vi "Cron&EventTab@ShortcutsStart__Parameter.vi"(1 "ParamterIn":string) -> (0 "ParamterOut":string)   [LabVIEW 2020]
panel:
  in  "Conditioin":string
  in  "EventTabName":string(combo)
  in  "Confirm":bool
  # "Cron&EventTab@ShortcutsStart $ShortcutsTabName, $Key"
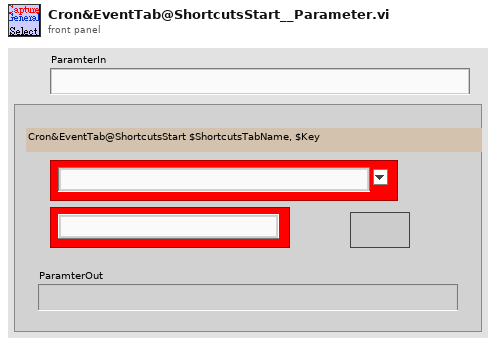
[diagram p1: front panel]
types:
  T1 = enum16{"Init", "Add", "Enable", "Disable", "Get"}
  T2 = cluster{"Shift":bool, "Ctrl":bool, "Alt":bool, "Cmd":bool, "Opt":bool}
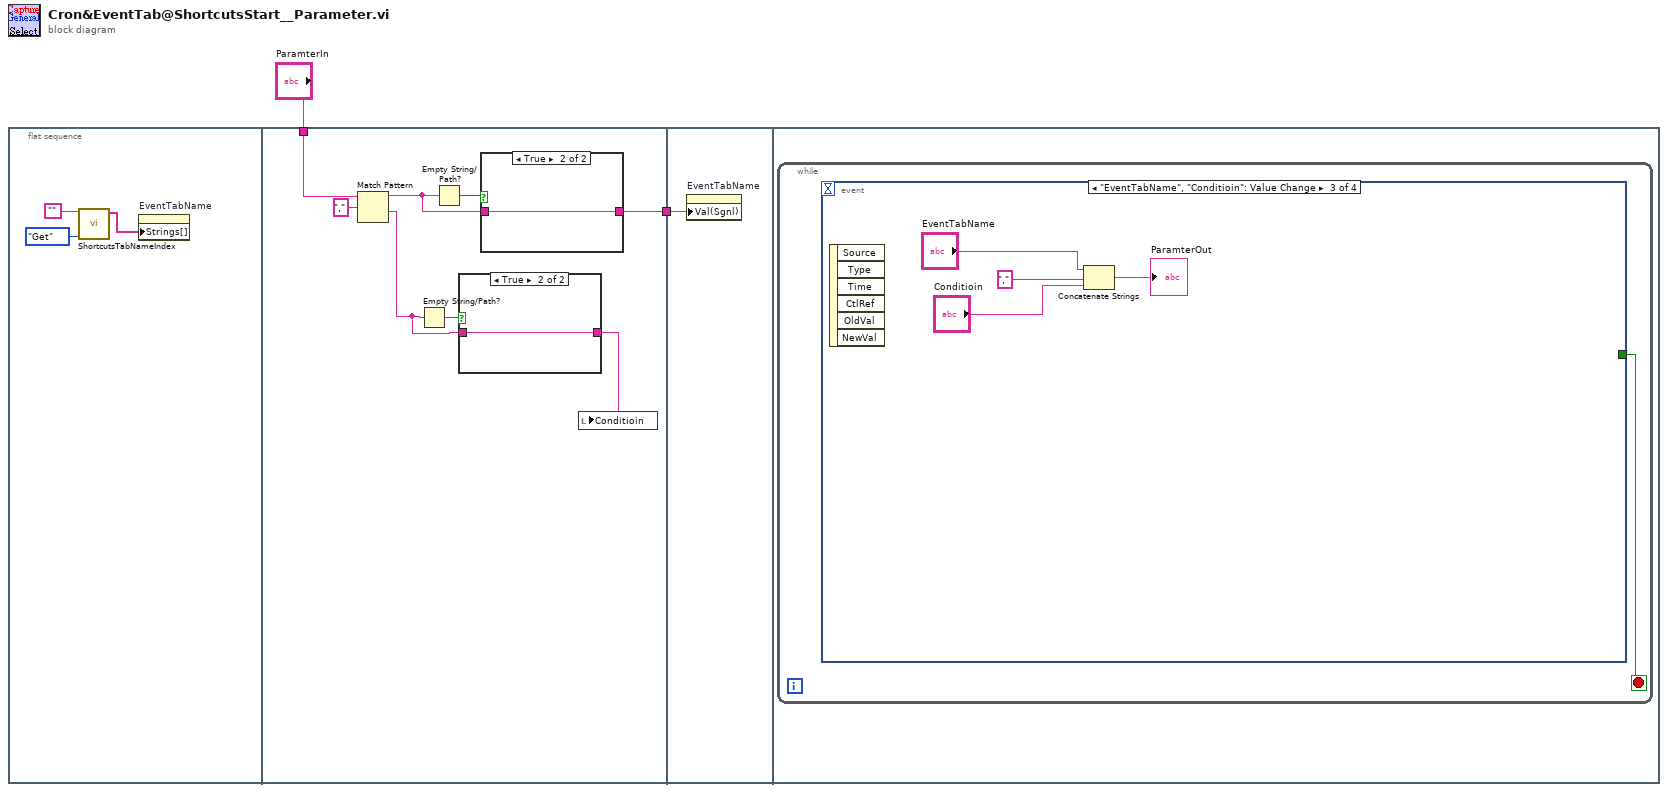
[diagram p0: block diagram]
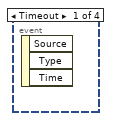
[diagram p4: hidden frame]
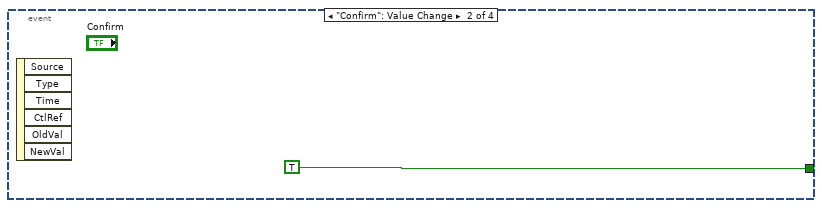
[diagram p5: hidden frame]
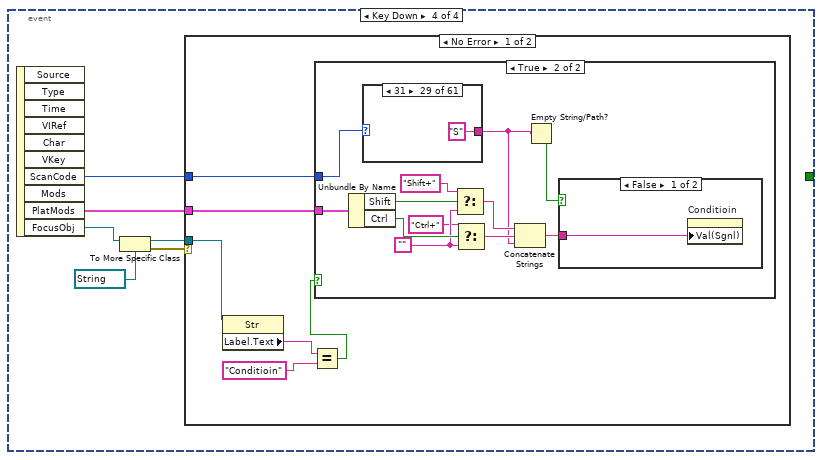
[diagram p6: hidden frame]
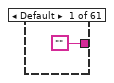
[diagram p9: hidden frame]
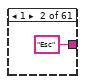
[diagram p10: hidden frame]
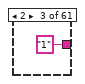
[diagram p11: hidden frame]
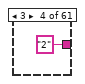
[diagram p12: hidden frame]
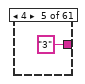
[diagram p13: hidden frame]
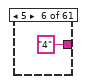
[diagram p14: hidden frame]
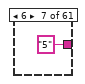
[diagram p15: hidden frame]
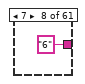
[diagram p16: hidden frame]
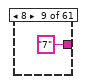
[diagram p17: hidden frame]
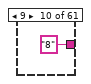
[diagram p18: hidden frame]
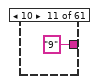
[diagram p19: hidden frame]
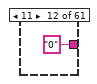
[diagram p20: hidden frame]
diagram:
  n1 = flat-sequence {
    tunnel: "ParamterIn" -> [w11]
    tunnel: [w12] -> w1
    tunnel: w1 -> [w18]
    frame #0 {
      n2 = call "ShortcutsTabNameIndex.vi"("OP"=T1."Get", "KeyTabName"="") -> ("KeyTabNameS"=w3:string[])  [unwired: 6 in, 3 out]
      n3 = property on="EventTabName" class="CmbBox"("Strings[]"=w3) -> ()  [unwired: 2 in, 2 out]
    }
    frame #1 {
      n4 = Match Pattern(string=w11, regular expression=",") -> (before substring=w9:string, after substring=w7:string)  [unwired: 1 in, 2 out]
      n5 = Empty String/Path?(string/path=w7) -> (empty?=w8:bool)
      n6 = Empty String/Path?(string/path=w9) -> (empty?=w13:bool)
      n7 = case shown="True" w8 {
        tunnel: w7 -> [w14 w15]
        tunnel: [w14 w15] -> w6
        frame False {
        }
        frame True {
        }
      }
      n8 = case shown="True" w13 {
        tunnel: w9 -> [w16 w17]
        tunnel: [w16 w17] -> w12
        frame False {
        }
        frame True {
        }
      }
      n9 = local write "Conditioin"(w6) -> ()
    }
    frame #2 {
      n10 = property on="EventTabName" class="CmbBox"("Val(Sgnl)"=w18) -> ()  [unwired: 2 in, 2 out]
    }
    frame #3 {
      n11 = while {
        stop <- w19 stop-if-true
        n12 = event shown="[2] \"EventTabName\", \"Conditioin\": Value Change" {
          selector: _ -> [_ _ _ _]
          dyn-events: _ -> [_ _ _ _]
          timeout: _ -> [_ _ _ _]
          tunnel: [_ TRUE _ _] -> w19
          event Timeout {
            n13 = event-data() -> ()  [unwired: 1 in, 3 out]
          }
          event "Confirm": Value Change {
            n14 = event-data() -> ()  [unwired: 1 in, 6 out]
          }
          event "EventTabName", "Conditioin": Value Change {
            n15 = event-data() -> ()  [unwired: 1 in, 6 out]
            n16 = Concatenate Strings("EventTabName", "," ("string"), "Conditioin") -> (→"ParamterOut":string)
          }
          event Key Down {
            n17 = event-data() -> ("ScanCode"=w29:i16, "PlatMods"=w30:T2, "FocusObj"=w28:refnum<vi>)  [unwired: 1 in, 7 out]
            n18 = To More Specific Class(target class=refnum<vi> refnum ("Conditioin"), reference=w28) -> (specific class reference=w26:refnum<vi>, error out=w27:errorcluster)  [unwired: 1 in]
            n19 = case shown="No Error" w27 {
              tunnel: w30 -> [w36 _]
              tunnel: w29 -> [w35 _]
              tunnel: w26 -> [w34 _]
              frame No Error {
                n20 = property class="Str"(reference=w34) -> ("Label.Text"=w33:string)  [unwired: 1 in, 2 out]
                n21 = Equal?(x=w33, y="Conditioin") -> (x = y?=w31:bool)
                n22 = case shown="True" w31 {
                  tunnel: w36 -> [_ w41]
                  tunnel: w35 -> [_ w40]
                  frame False {
                  }
                  frame True {
                    w44 = ""
                    n23 = Unbundle By Name(w41) -> ("Shift"=w45:bool, "Ctrl"=w46:bool)
                    n24 = case shown="31" w40 {
                      tunnel: ["" "Esc" "1" "2" "3" "4" "5" "6" "7" "8" "9" "0" "-" "=" "Q" "W" "E" "R" "T" "Y" "U" "I" "O" "P" "[" "]" "]" "A" "S" "D" "F" "G" "H" "J" "L" "Z" "X" "C" "V" "B" "N" "M" "<" ">" "?" "F2" "F3" "F4" "F5" "F6" "F7" "F8" "F9" "F10" "Home" "PageUp" "End" "PageDown" "Del" "F11" "F12"] -> w39
                      frame Default {
                      }
                      frame 1 {
                      }
                      frame 2 {
                      }
                      frame 3 {
                      }
                      frame 4 {
                      }
                      frame 5 {
                      }
                      frame 6 {
                      }
                      frame 7 {
                      }
                      frame 8 {
                      }
                      frame 9 {
                      }
                      frame 10 {
                      }
                      frame 11 {
                      }
                      frame 12 {
                      }
                      frame 13 {
                      }
                      frame 16 {
                      }
                      frame 17 {
                      }
                      frame 18 {
                      }
                      frame 19 {
                      }
                      frame 20 {
                      }
                      frame 21 {
                      }
                      frame 22 {
                      }
                      frame 23 {
                      }
                      frame 24 {
                      }
                      frame 25 {
                      }
                      frame 26 {
                      }
                      frame 27 {
                      }
                      frame 28 {
                      }
                      frame 30 {
                      }
                      frame 31 {
                      }
                      frame 32 {
                      }
                      frame 33 {
                      }
                      frame 34 {
                      }
                      frame 35 {
                      }
                      frame 36 {
                      }
                      frame 37 {
                      }
                      frame 44 {
                      }
                      frame 45 {
                      }
                      frame 46 {
                      }
                      frame 47 {
                      }
                      frame 48 {
                      }
                      frame 49 {
                      }
                      frame 50 {
                      }
                      frame 51 {
                      }
                      frame 52 {
                      }
                      frame 53 {
                      }
                      frame 60 {
                      }
                      frame 61 {
                      }
                      frame 62 {
                      }
                      frame 63 {
                      }
                      frame 64 {
                      }
                      frame 65 {
                      }
                      frame 66 {
                      }
                      frame 67 {
                      }
                      frame 68 {
                      }
                      frame 71 {
                      }
                      frame 73 {
                      }
                      frame 79 {
                      }
                      frame 81 {
                      }
                      frame 83 {
                      }
                      frame 87 {
                      }
                      frame 88 {
                      }
                    }
                    n25 = Select(t="Shift+", s=w45, f=w44) -> (s? t:f=w47:string)
                    n26 = Select(t="Ctrl+", s=w46, f=w44) -> (s? t:f=w48:string)
                    n27 = Concatenate Strings(w47, w48, w39) -> (w37:string)
                    n28 = Empty String/Path?(string/path=w39) -> (empty?=w38:bool)
                    n29 = case shown="False" w38 {
                      tunnel: w37 -> [w49 _]
                      frame False {
                        n30 = property on="Conditioin" class="Str"("Val(Sgnl)"=w49) -> ()  [unwired: 2 in, 2 out]
                      }
                      frame True {
                      }
                    }
                  }
                }
              }
              frame Error {
              }
            }
          }
        }
      }
    }
  }
